vi "Ethernet IP Custom Device RT Driver VI.vi"(6 "Device Clock":string, 9 "Device Inputs FIFO":refnum<k33>, 10 "Device Outputs FIFO":refnum<k33>, 11 "Device Reference":T1 format="%.0x") -> ()   [LabVIEW 2011, in "Ethernet IP Custom Device Custom Device.lvlib"]
uses:
  Ethernet IP Custom Device Custom Device.lvlib
  <vilib>/NI Veristand/Custom Device API/Custom Device Item Ref.ctl
  <vilib>/NI Veristand/Custom Device API/Custom Device Channel Type.ctl
  <vilib>/Platform/TimedLoop/XDataNode/timing_clust.ctl
  <vilib>/Platform/TimedLoop/XDataNode/nitl_modes.ctl
  <vilib>/Platform/TimedLoop/XDataNode/wakeup.ctl
  Ethernet IP Global Strings.vi
  <vilib>/NI Veristand/Custom Device API/Get Item Property (I32).vi
  <vilib>/NI Veristand/Custom Device API/Get Item Property (String).vi
  <vilib>/ethernetip/ethernetip.llb/EthernetIP Tag Write.vi
  <vilib>/ethernetip/ethernetip.llb/EthernetIP Tag Write SINT.vi
  <vilib>/ethernetip/ethernetip.llb/EthernetIP Tag Write INT.vi
  <vilib>/ethernetip/ethernetip.llb/EthernetIP Tag Write DINT.vi
  <vilib>/ethernetip/ethernetip.llb/EthernetIP Tag Write REAL.vi
  <vilib>/ethernetip/ethernetip.llb/EthernetIP Tag Write BOOL.vi
  <vilib>/ethernetip/ethernetip.llb/EthernetIP Tag Read.vi
  <vilib>/ethernetip/ethernetip.llb/EthernetIP Tag Read INT.vi
  <vilib>/ethernetip/ethernetip.llb/EthernetIP Tag Read DINT.vi
  <vilib>/ethernetip/ethernetip.llb/EthernetIP Tag Read REAL.vi
  <vilib>/ethernetip/ethernetip.llb/EthernetIP Tag Read BOOL.vi
  <vilib>/ethernetip/ethernetip.llb/EthernetIP Tag Read SINT.vi
  <vilib>/Platform/TimedLoop/XDataNode/XDataNode.xnode
  <vilib>/Platform/TimedLoop/XDataNode/XDNodeRunTimeDep.lvlib
  <vilib>/NI Veristand/Custom Device API/Custom Device API.lvlib
  <vilib>/NI Veristand/Custom Device Tools/Custom Device Utility Library/Custom Device Utility Library.lvlib
  <vilib>/ethernetip/ethernetip.lvlib
panel:
  in  "Initialization Status Notifier":refnum<notifier>
  in  "Status Notifier":refnum<notifier>
  # "Custom Device Template\nv1.0"
  # "Use this template as a starting point for creating a custom device code module. The input controls shown here are specially named controls that the system will use to provide the device loop with data. The controls are not required for the device loop to run. For instance, if the device doesn't produce any output data, then you don't need the Device Outputs FIFO control. If you do use these controls, however, they need to have these exact names to be functional."
  # "The optional status notifier element is used to notify the RT engine of the last state of the custom device, and to indicate the device has completed execution. If this control is not used, a default No Error value is returned to the system when the device finishes execution.\n\nNote: This error state is not checked until the system shuts down. Use an output status channel to send more immediate status values to the system."
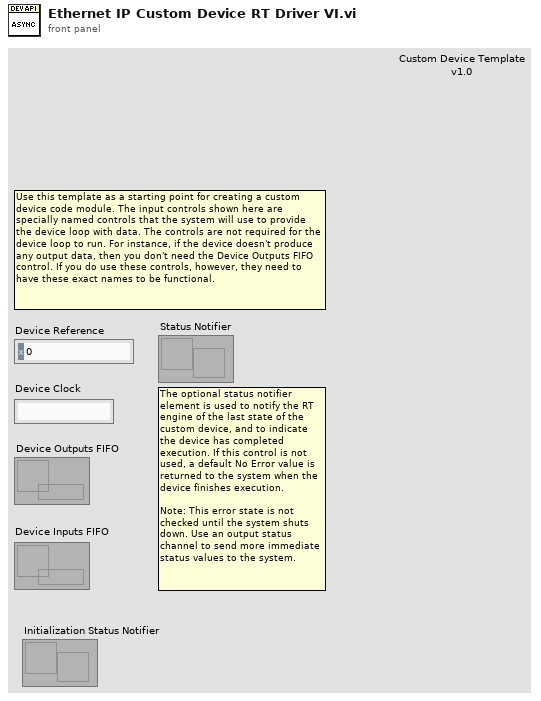
[diagram p1: front panel]
types:
  T1 = typedef "Custom Device API.lvlib/Custom Device Item Ref.ctl" = u64
  T2 = typedef "Custom Device API.lvlib/Custom Device Channel Type.ctl" = enum16{"Input", "Output"}
  T3 = typedef "Custom Device API.lvlib/Custom Device Timed Loop Priority.ctl" = enum32{"Low", "Medium", "High"}
  T4 = typedef "Custom Device API.lvlib/Custom Device Item Info.ctl" = cluster{"Name":string, "Is Channel":bool, "GUID":string}
  T5 = typedef "Ethernet IP Custom Device Custom Device.lvlib/EIP Tag Information.ctl" = cluster{"Item Info":T4, "Device Reference":T1, "Channel Indices":i32[], "Tag Name":string, "Data Type":T6}
  T6 = typedef "Ethernet IP Custom Device Custom Device.lvlib/L5K Data Types.ctl" = enum16{"SINT", "INT", "DINT", "REAL", "BOOL"}
  T7 = typedef "ethernetip.lvlib/ethernetip.ctl" = refnum<k21>
  T8 = typedef "XDNodeRunTimeDep.lvlib/timing_clust.ctl" = cluster{"Expected End [f-1]":u64, "Actual End [f-1]":u64, "Finished Late? [f-1]":bool, "Expected End [i-1]":u64, "Actual End [i-1]":u64, "Finished Late? [i-1]":bool, "Expected Start [i]":u64, "Actual Start [i]":u64, "Expected Start [f]":u64, "Actual Start [f]":u64, "Source Name":string, "Structure Name":string, "Period":i64, "Deadline":i64, "Offset":i64, "Start":i64, "Priority":i32, "Timeout":i32, "Mode":T9, "Wakeup Reason":T10, "Error":errorcluster, "Source Type":string, "Secondary Source Type":string, "Global End Time":u64, "Global Start Time":u64, "Frame Duration":u64, "Iteration Duration":u64, "Assigned CPU":i32, "I/O Scan Engine Mode":u32}
  T9 = typedef "XDNodeRunTimeDep.lvlib/nitl_modes.ctl" = enum32{"No Change", "Process missed periods, maintain original phase", "Discard missed periods, maintain original phase", "Process missed periods, ignore original phase", "Discard missed periods, ignore original phase"}
  T10 = typedef "XDNodeRunTimeDep.lvlib/wakeup.ctl" = enum32{"Normal", "Aborted", "Asynchronous wakeup", "Timing source error", "Timed loop error", "Timeout"}
  T11 = typedef "Ethernet IP Custom Device Custom Device.lvlib/EIP Device Settings.ctl" = cluster{"Path":string, "Timeout":i32}
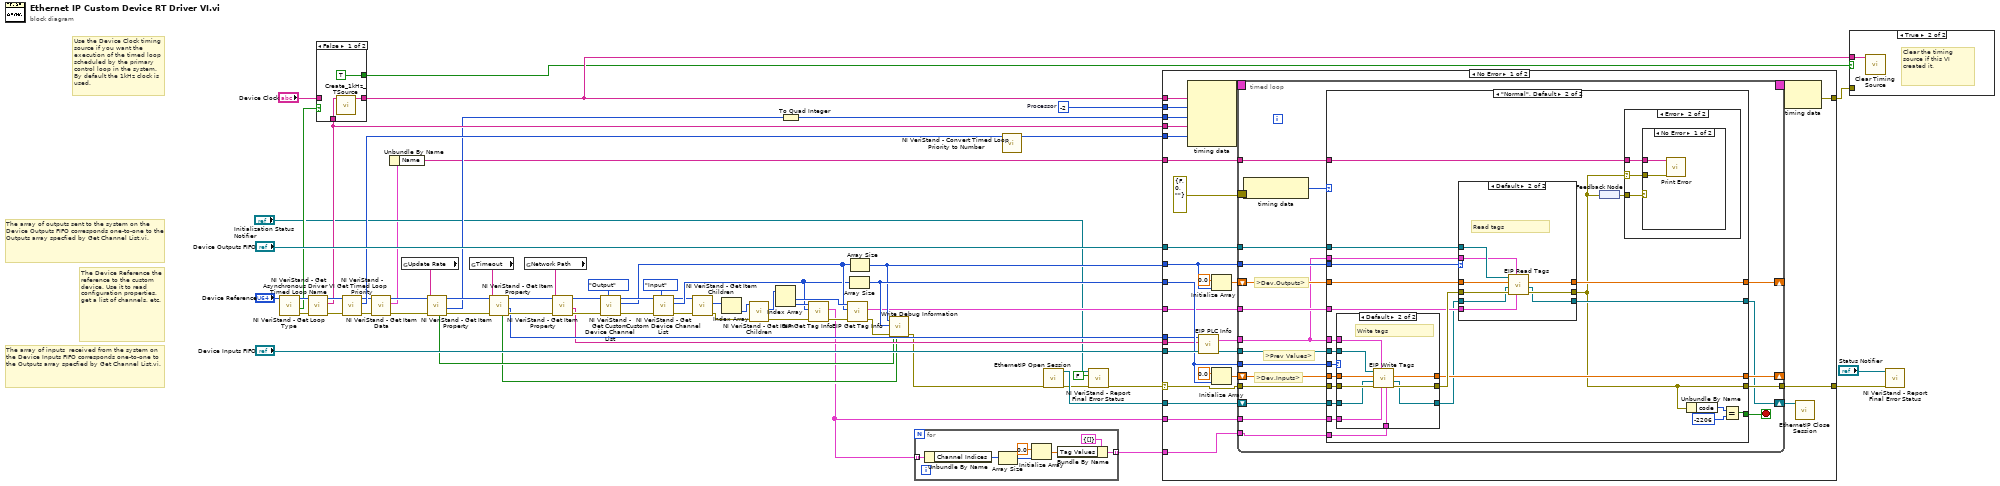
[diagram p0: block diagram]
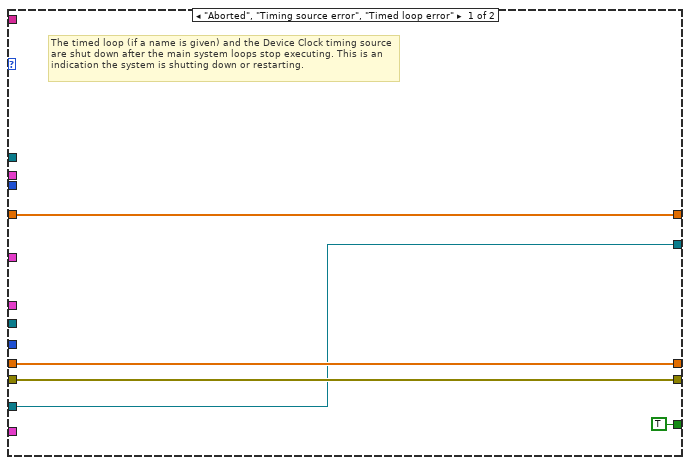
[diagram p2: hidden frame]
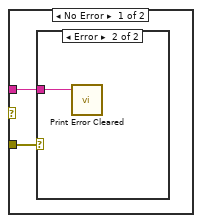
[diagram p3: hidden frame]
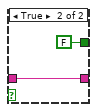
[diagram p10: hidden frame]
diagram:
  w57 = -2  # Processor
  # "The array of inputs  received from the system on the Device Inputs FIFO corresponds one-to-one to the Outputs array specfied by Get Channel List.vi."
  # "The array of outputs sent to the system on the Device Outputs FIFO corresponds one-to-one to the Outputs array specfied by Get Channel List.vi."
  # "The Device Reference the reference to the custom device. Use it to read configuration properties, get a list of channels, etc."
  # "Use the Device Clock timing source if you want the execution of the timed loop scheduled by the primary control loop in the system. \nBy default the 1kHz clock is used."
  n1 = call <vilib>:"NI VeriStand - Get Loop Type.vi"("Device Ref in"="Device Reference") -> ("error out"=w56:errorcluster, "Use Device Clock"=w53:bool, "Device Ref out"=w55:T1)  [unwired: 1 in, 7 out]
  n2 = call <vilib>:"NI VeriStand - Get Asynchronous Driver VI Timed Loop Name.vi"("error in (no error)"=w56, "Device Ref in"=w55) -> ("error out"=w60:errorcluster, "Device Timed Loop Name"=w48:string, "Device Ref out"=w67:T1)  [unwired: 7 out]
  n3 = case shown="False" w53 {
    tunnel: "Device Clock" -> [_ w72]
    tunnel: [w70 w72] -> w49
    tunnel: [TRUE FALSE] -> w20
    tunnel: w48 -> [w68 _]
    frame False {
      n4 = call <vilib>:"Create_1kHz_TSource.vi"("name (in)"=w68) -> ("name (out)"=w70:string)  [unwired: 1 in, 9 out]
    }
    frame True {
    }
  }
  n5 = call <vilib>:"NI VeriStand - Get Timed Loop Priority.vi"("error in (no error)"=w60, "Device Ref in"=w67) -> ("error out"=w26:errorcluster, "Priority"=w59:T3, "Device Ref out"=w4:T1)  [unwired: 7 out]
  n6 = call <vilib>:"NI VeriStand - Get Item Data.vi"("error in (no error)"=w26, "Item Ref in"=w4) -> ("error out"=w5:errorcluster, "Item Info"=w2:T4, "Item Ref out"=w3:T1)  [unwired: 6 in, 1 out]
  n7 = Unbundle By Name(w2) -> ("Name"=w1:string)
  n8 = global read "Ethernet IP Global Strings.vi" "Update Rate"() -> (w24:string)
  n9 = call-poly <vilib>:"NI VeriStand - Get Item Property.vi"("error in (no error)"=w5, "Property Name"=w24, "Item Ref in"=w3) -> ("error out"=w32:errorcluster, "Value"=w21:i32, "Item Ref out"=w30:T1, "Found?"=w13:bool)  [unwired: 5 in]
  n10 = global read "Ethernet IP Global Strings.vi" "Timeout"() -> (w27:string)
  n11 = call-poly <vilib>:"NI VeriStand - Get Item Property.vi"("error in (no error)"=w32, "Property Name"=w27, "Item Ref in"=w30) -> ("error out"=w31:errorcluster, "Value"=w18:i32, "Item Ref out"=w29:T1, "Found?"=w12:bool)  [unwired: 5 in]
  n12 = global read "Ethernet IP Global Strings.vi" "Network Path"() -> (w28:string)
  n13 = call-poly <vilib>:"NI VeriStand - Get Item Property.vi"("error in (no error)"=w31, "Property Name"=w28, "Item Ref in"=w29) -> ("error out"=w25:errorcluster, "Value"=w17:string, "Item Ref out"=w22:T1)  [unwired: 5 in, 1 out]
  n14 = call <vilib>:"NI VeriStand - Get Custom Device Channel List.vi"("Channel Type"=Custom_Device_Channel_Type."Output", "error in (no error)"=w25, "Device Ref in"=w22) -> ("error out"=w62:errorcluster, "Specified Channel Ref List"=w44:T1[], "Device Ref out"=w63:T1)  [unwired: 6 out]
  n15 = call <vilib>:"NI VeriStand - Get Custom Device Channel List.vi"("Channel Type"=Custom_Device_Channel_Type."Input", "error in (no error)"=w62, "Device Ref in"=w63) -> ("error out"=w33:errorcluster, "Specified Channel Ref List"=w43:T1[], "Device Ref out"=w34:T1)  [unwired: 6 out]
  n16 = call <vilib>:"NI VeriStand - Get Item Children.vi"("error in (no error)"=w33, "Item Ref in"=w34) -> ("error out"=w42:errorcluster, "Child Refs"=w40:T1[])  [unwired: 6 in, 2 out]
  n17 = Index Array(array=w40) -> (element=w39:T1)  [unwired: 1 in]
  n18 = call <vilib>:"NI VeriStand - Get Item Children.vi"("error in (no error)"=w42, "Item Ref in"=w39) -> ("error out"=w41:errorcluster, "Child Refs"=w38:T1[])  [unwired: 6 in, 2 out]
  n19 = Index Array(array=w38) -> (element #1=w46:T1, element #2=w45:T1)  [unwired: 2 in]
  n20 = To Quad Integer(1:w21) -> (0:w37:i64)
  n21 = call "EIP Get Tag Info.vi"("error in"=w41, "Specified Channel Ref List"=w43, "Item Ref in"=w45) -> ("error out"=w47:errorcluster, "Tag Data"=w11:T5[])  [unwired: 6 in, 1 out]
  n22 = call "EIP Get Tag Info.vi"("error in"=w47, "Specified Channel Ref List"=w44, "Item Ref in"=w46) -> ("error out"=w23:errorcluster, "Tag Data"=w15:T5[])  [unwired: 6 in, 1 out]
  n23 = Array Size(array=w43) -> (size(s)=w19:i32)
  n24 = Array Size(array=w44) -> (size(s)=w16:i32)
  n25 = call "Write Debug Information.vi"("Timeout Property found?"=w12, "Update Property Found?"=w13, "error in"=w23, "Tags to write"=w19, "Tags to read"=w16) -> ("error out"=w14:errorcluster)  [unwired: 5 in, 1 out]
  n26 = for {
    tunnel: w11 -> [w79] mode=indexing
    tunnel: [w73] -> w10 mode=indexing
    n27 = Unbundle By Name(w79) -> ("Channel Indices"=w78:i32[])
    n28 = Array Size(array=w78) -> (size(s)=w76:i32)
    n29 = Initialize Array(0.0, w76) -> (w74:dbl[])
    n30 = Bundle By Name(cluster=cluster{"Tag Values":dbl[]} {"Tag Values"=[]} ("Tag Values"), "Tag Values"=w74) -> (w73:cluster{"Tag Values":dbl[]})
  }
  n31 = call <vilib>:"NI VeriStand - Convert Timed Loop Priority to Number.vi"("Priority"=w59) -> ("Numeric Priority"=w58:i32)  [unwired: 10 out]
  n32 = call <vilib>:"EthernetIP Open Session.vi"("error in"=w14) -> ("error out"=w9:errorcluster, "Session out"=w36:T7)  [unwired: 9 in]
  n33 = call <vilib>:"NI VeriStand - Report Final Error Status.vi"("error in (no error)"=w9, "Filter FIFO Errors (T)"=FALSE, "Status Notifier"="Initialization Status Notifier") -> ("error out"=w6:errorcluster)  [unwired: 8 out]
  n34 = case shown="No Error" w6 {
    selector: w6 -> [w83 w201]
    tunnel: "Device Outputs FIFO" -> [w105 _]
    tunnel: "Device Inputs FIFO" -> [w104 _]
    tunnel: w58 -> [w100 _]
    tunnel: w57 -> [w99 _]
    tunnel: [w98 _] -> w50
    tunnel: w49 -> [w97 _]
    tunnel: w48 -> [w96 _]
    tunnel: w37 -> [w94 _]
    tunnel: w36 -> [w93 _]
    tunnel: [w80 w201] -> w35
    tunnel: w19 -> [w91 _]
    tunnel: w18 -> [w90 _]
    tunnel: w17 -> [w89 _]
    tunnel: w16 -> [w88 _]
    tunnel: w15 -> [w87 _]
    tunnel: w11 -> [w85 _]
    tunnel: w10 -> [w84 _]
    tunnel: w1 -> [w81 _]
    frame No Error {
      n35 = node-c288(w97, w99, w94, w96, w100) -> (w107:T8)
      n36 = call "EIP PLC Info.vi"("Path"=w89, "Timeout"=w90) -> ("Device Settings"=w95:T11)  [unwired: 5 in]
      n37 = Initialize Array(0.0 ("element"), w88) -> (w101:dbl[])
      n38 = Initialize Array(0.0 ("element"), w91) -> (w86:dbl[])
      n39 = timed-loop {
        timing: w107 -> [_]
        timing-out: [_] -> w106
        shift-right: [w124] -> _
        shift-left: w86 -> [w125]
        shift-right: [w122] -> _
        shift-left: w101 -> [w123]
        tunnel: w88 -> [w119]
        tunnel: w105 -> [w121]
        tunnel: w104 -> [w120]
        tunnel: w91 -> [w117]
        tunnel: w87 -> [w115]
        tunnel: w85 -> [w116]
        tunnel: w95 -> [w114]
        shift-right: [w112] -> w92
        shift-left: w93 -> [w113]
        tunnel: w84 -> [w111]
        tunnel: w83 -> [w126]
        tunnel: [w118] -> w80
        border: errorcluster {"status"=FALSE, "code"=0, "source"=""} ("error out") -> [_]
        tunnel: w81 -> [w108]
        stop <- w109 stop-if-true
        # ">Prev Values>"
        # ">Dev.Outputs>"
        # ">Dev.Inputs>"
        n40 = node-c288() -> (w110:T10)  [unwired: 1 out]
        n41 = case shown="\"Normal\", Default" w110 {
          tunnel: w126 -> [w130 w150]
          tunnel: w125 -> [w131 w152]
          tunnel: [w130 w133] -> w118
          tunnel: [w131 w146] -> w124
          tunnel: w123 -> [w129 w153]
          tunnel: [w129 w151] -> w122
          tunnel: w121 -> [_ w155]
          tunnel: w120 -> [_ w154]
          tunnel: w119 -> [_ w148]
          tunnel: [TRUE w132] -> w109
          tunnel: w117 -> [_ w149]
          tunnel: w116 -> [_ w145]
          tunnel: w115 -> [_ w144]
          tunnel: w114 -> [_ w143]
          tunnel: w114 -> [_ w142]
          tunnel: w113 -> [w127 w141]
          tunnel: [w127 w139] -> w112
          tunnel: w111 -> [_ w138]
          tunnel: w108 -> [_ w136]
          frame "Aborted", "Timing source error", "Timed loop error" {
            # "The timed loop (if a name is given) and the Device Clock timing source are shut down after the main system loops stop executing. This is an indication the system is shutting down or restarting."
          }
          frame "Normal", Default {
            n42 = case shown="Default" w149 {
              tunnel: w154 -> [_ w188]
              tunnel: w152 -> [w178 w184]
              tunnel: [w178 w185] -> w146
              tunnel: [w177 w186] -> w147
              tunnel: w150 -> [w177 w187]
              tunnel: w145 -> [_ w183]
              tunnel: w143 -> [_ w182]
              tunnel: w141 -> [w176 w181]
              tunnel: [w176 w180] -> w140
              tunnel: w138 -> [_ w179]
              frame 0 {
                # "No inputs to read\nfrom system. Inputs FIFO not created in this case, so don't write to it."
              }
              frame Default {
                # "Write tags"
                n43 = call "EIP Write Tags.vi"("Previous Values buffer"=w179, "Tag Data"=w183, "Device Settings"=w182, "error in"=w187, "Session In"=w181, "Device Inputs In"=w184, "Device Inputs FIFO"=w188) -> ("error out"=w186:errorcluster, "Session Out"=w180:T7, "Device Inputs Out"=w185:dbl[])  [unwired: 2 in]
              }
            }
            n44 = case shown="Default" w148 {
              tunnel: w155 -> [_ w174]
              tunnel: w153 -> [w166 w175]
              tunnel: [w166 w173] -> w151
              tunnel: w147 -> [w165 w172]
              tunnel: [w165 w171] -> w133
              tunnel: w144 -> [_ w170]
              tunnel: w142 -> [_ w169]
              tunnel: w140 -> [w164 w168]
              tunnel: [w164 w167] -> w139
              frame 0 {
                # "No outputs to write to system. \nThe Device Outputs FIFO\nis never created in this case,\nso don't write to it."
              }
              frame Default {
                # "Read tags"
                n45 = call "EIP Read Tags.vi"("Tag Data"=w170, "Device Settings"=w169, "error in"=w172, "Session In"=w168, "Device Outputs In"=w175, "Device Outputs FIFO"=w174) -> ("error out"=w171:errorcluster, "Session Out"=w167:T7, "Device Outputs Out"=w173:dbl[])  [unwired: 3 in]
              }
            }
            n46 = feedback-in #1(w133) -> ()
            n47 = feedback #1() -> (w137:errorcluster)
            n48 = case shown="Error" w133 {
              selector: w133 -> [_ w160]
              tunnel: w137 -> [w157 w161]
              tunnel: w136 -> [w156 w159]
              frame No Error {
                n49 = case shown="Error" w157 {
                  tunnel: w156 -> [_ w158]
                  frame No Error {
                  }
                  frame Error {
                    n50 = call "Print Error Cleared.vi"("Your code's public name"=w158) -> ()  [unwired: 10 in]
                  }
                }
              }
              frame Error {
                n51 = case shown="No Error" w161 {
                  tunnel: w160 -> [w163 _]
                  tunnel: w159 -> [w162 _]
                  frame No Error {
                    n52 = call "Print Error.vi"("error out"=w163, "Your code's public name"=w162) -> ()  [unwired: 10 in]
                  }
                  frame Error {
                  }
                }
              }
            }
            n53 = Unbundle By Name(w133) -> ("code"=w135:i32)
            n54 = Equal?(x=w135, y=-2206) -> (x = y?=w132:bool)
          }
        }
      }
      n55 = node-c288(w106) -> (w98:errorcluster)
      n56 = call <vilib>:"EthernetIP Close Session.vi"("Session in"=w92) -> ()  [unwired: 10 in, 1 out]
    }
    frame Error {
    }
  }
  n57 = case shown="True" w20 {
    tunnel: w50 -> [_ _]
    tunnel: w49 -> [_ w202]
    frame False {
    }
    frame True {
      # "Clear the timing source if this VI created it."
      n58 = call <vilib>:"Clear Timing Source.vi"("name"=w202) -> ()  [unwired: 1 in, 10 out]
    }
  }
  n59 = call <vilib>:"NI VeriStand - Report Final Error Status.vi"("error in (no error)"=w35, "Status Notifier"="Status Notifier") -> ()  [unwired: 1 in, 9 out]
